vi "Open Document.vi"(7 "Document Type":refnum<class "npoiDocument.lvclass">, 8 "error in (no error)":errorcluster, 11 "Document Path":path) -> (0 "error out":errorcluster, 3 "Document out":refnum<class "npoiDocument.lvclass">)   [LabVIEW 2017, in "NPOI_Document.lvlib" / "npoiDocument.lvclass"]
doc: "Opens an existing <b>Document out</b>,of the <b>Document Type</b> file format, at the <b>Document Path</b> location. Use save to persist your changes.\n\nNotes:\n - If <b>Document Path</b> is empty (default) or is <Not A Path> or is a directory, the VI displays a dialog box from which the user can select a file. Error 43 occurs if you cancel the dialog box."
uses:
  npoiDocument.lvclass
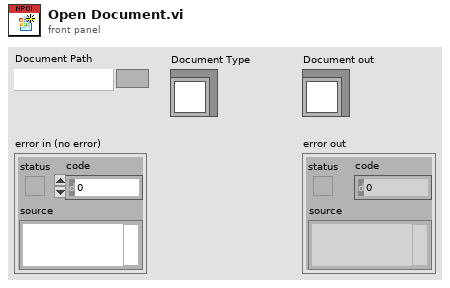
[diagram p1: front panel]
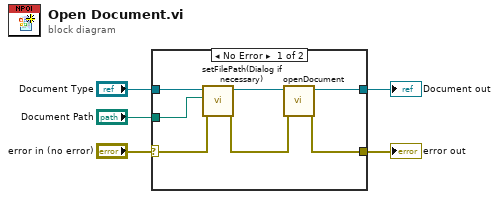
[diagram p0: block diagram]
diagram:
  n1 = case shown="No Error" "error in (no error)" {
    selector: "error in (no error)" -> [w7 w14]
    tunnel: [w11 w14] -> w4
    tunnel: [w12 w13] -> w2
    tunnel: "Document Type" -> [w10 w13]
    tunnel: "Document Path" -> [w8 _]
    frame No Error {
      n2 = call "setFilePath(Dialog if necessary).vi"("error in (no error)"=w7, "File Path"=w8, "npoiDocument in"=w10) -> ("error out"=w6:errorcluster, "npoiDocument out"=w9:refnum<class "npoiDocument.lvclass">)  [unwired: 7 in]
      n3 = call-dynamic "openDocument.vi"("error in (no error)"=w6, "npoiDocument in"=w9) -> ("error out"=w11:errorcluster, "npoiDocument out"=w12:refnum<class "npoiDocument.lvclass">)  [unwired: 8 in]
    }
    frame Error {
    }
  }
  "error out" <- w4
  "Document out" <- w2
